vi "Main.vi"() -> ()   [LabVIEW 2019]
panel:
  out "Main Tabs":T1(tab)
  in  "START GAME":bool
  in  "EXPERT SELECT":bool
  in  "HARD SELECT":bool
  in  "MEDIUM SELECT":bool
  in  "EASY SELECT":bool
  in  "EASY CODE":T2
  in  "SUBMIT EASY CODE":bool
  in  "MEDIUM CODE":T3
  in  "SUBMIT MEDIUM CODE":bool
  in  "HARD CODE":T3
  in  "SUBMIT HARD CODE":bool
  in  "EXPERT CODE":cluster{"A":u8, "B":u8, "C":u8, "D":u8}
  in  "SUBMIT EXPERT CODE":bool
  # "You have 5 minutes to solve a puzzle and escape.\nSelect your difficulty below:"
  # "Using the items on the table to your left\nfind and enter the code below"
  # "Solve the puzzle on the table to your right\nto find the code to escape"
  # "Interpret my speech with the key from the walls to open the codex.\nThen go to the table behind you to enter my song below"
  # "Use the panels around the room to tell me\nwhat number each letter represents"
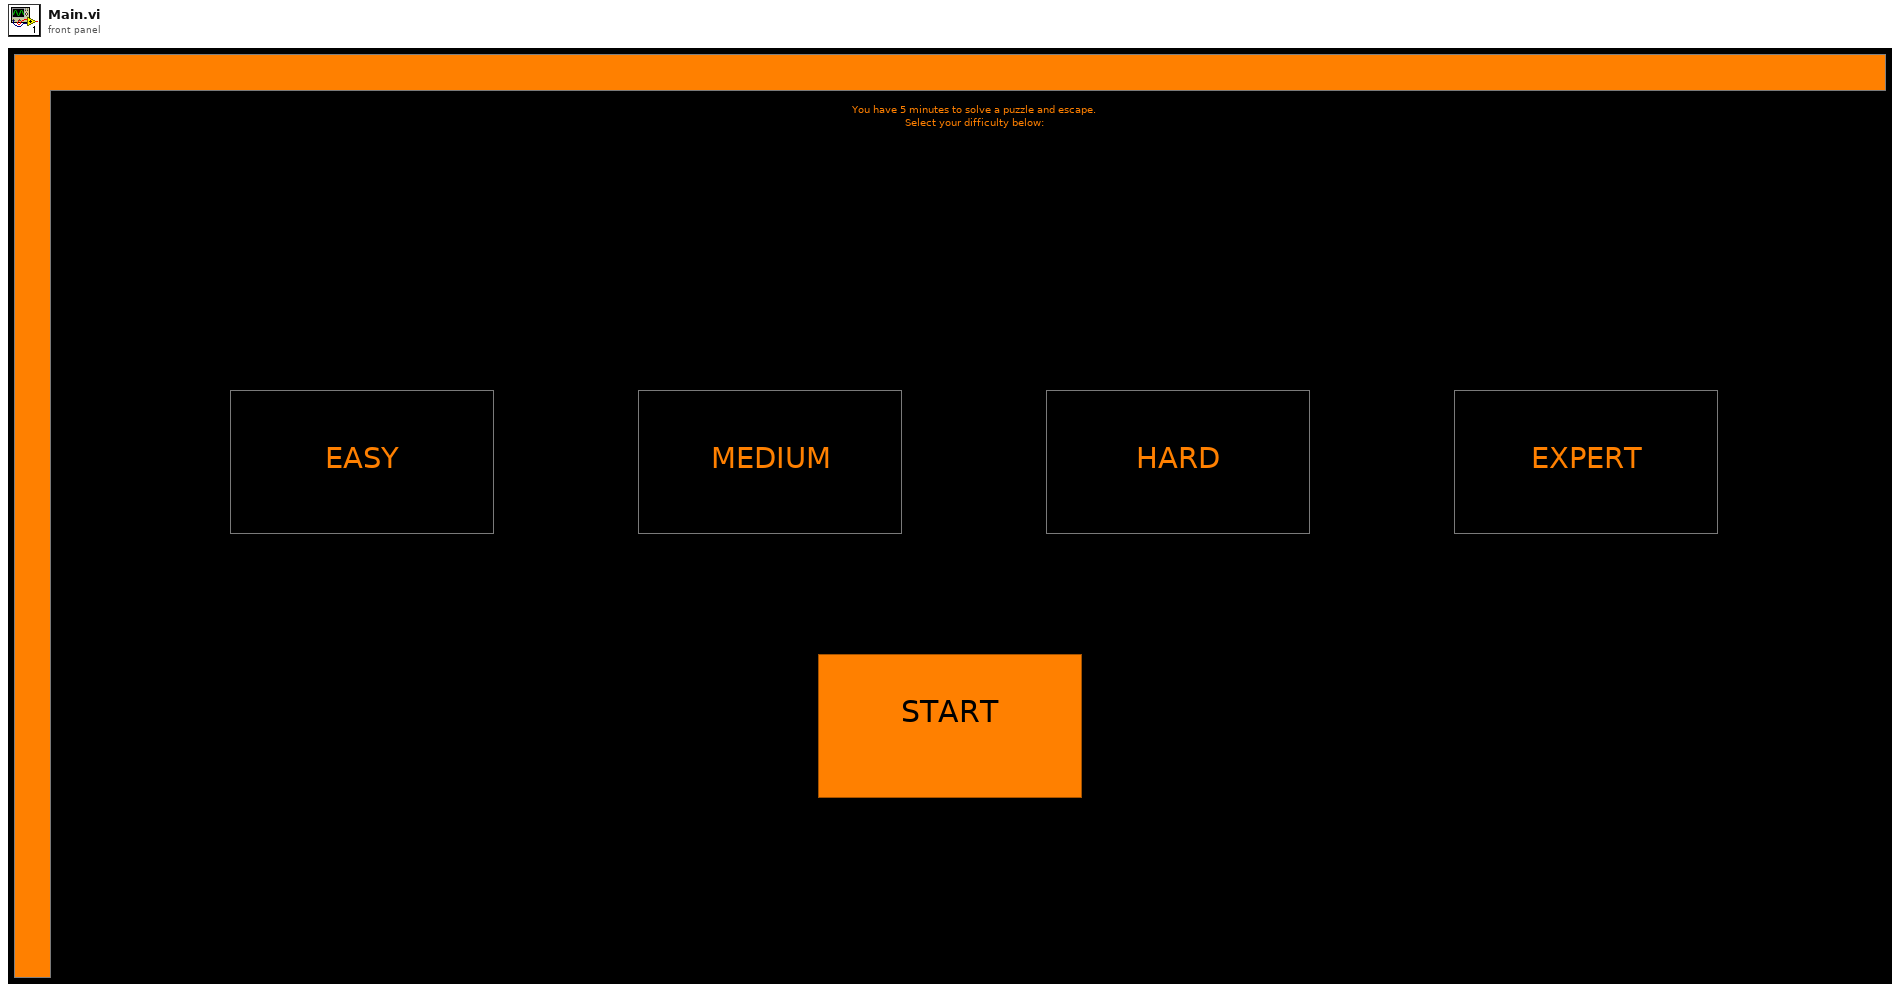
[diagram p1: front panel]
types:
  T1 = enum32{"START", "EASY", "MEDIUM", "HARD", "EXPERT", "END"}
  T2 = cluster{"CRANK":u8, "UV":u8, "MAZE":u8, "SCALE":u8}
  T3 = cluster{"DIGIT 1":u8, "DIGIT 2":u8, "DIGIT 3":u8, "DIGIT 4":u8}
  T4 = enum16{"INIT", "WAIT TO START", "GAME", "RESET", "END"}
  T5 = cluster{"CRANK":bool, "UV":bool, "MAZE":bool, "SCALE":bool}
  T6 = cluster{"DIGIT 1":bool, "DIGIT 2":bool, "DIGIT 3":bool, "DIGIT 4":bool}
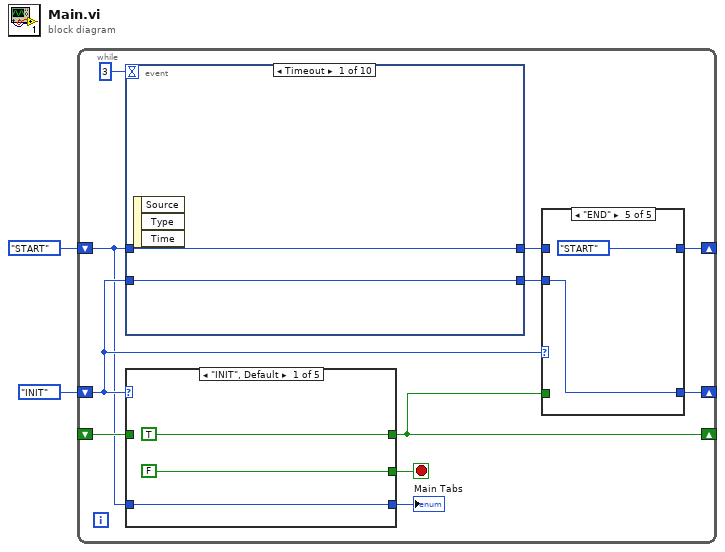
[diagram p0: block diagram]
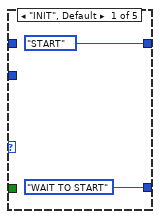
[diagram p2: hidden frame]
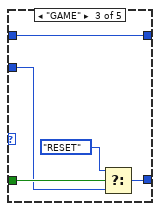
[diagram p4: hidden frame]
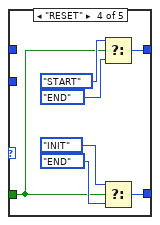
[diagram p5: hidden frame]
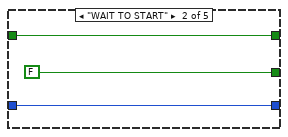
[diagram p6: hidden frame]
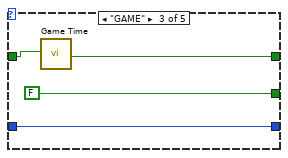
[diagram p7: hidden frame]
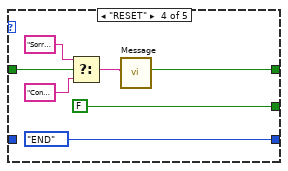
[diagram p8: hidden frame]
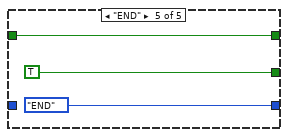
[diagram p9: hidden frame]
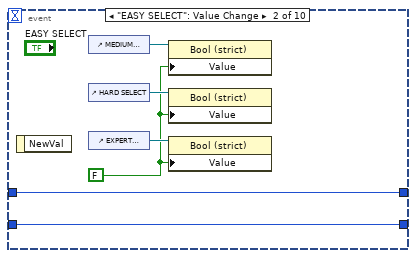
[diagram p10: hidden frame]
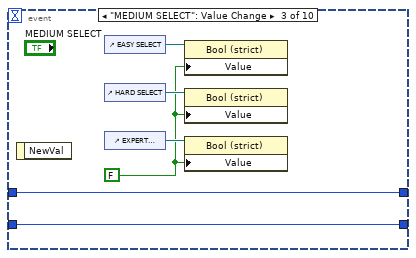
[diagram p11: hidden frame]
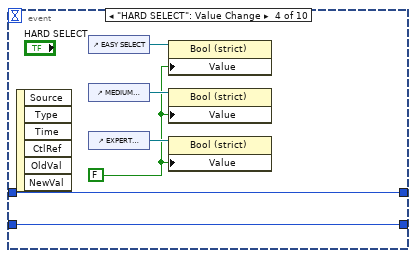
[diagram p12: hidden frame]
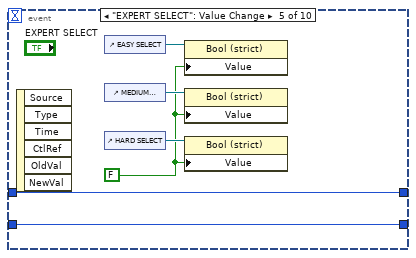
[diagram p13: hidden frame]
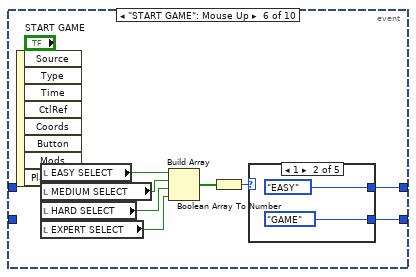
[diagram p14: hidden frame]
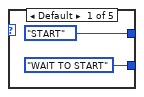
[diagram p15: hidden frame]
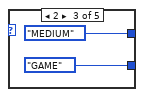
[diagram p16: hidden frame]
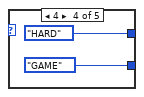
[diagram p17: hidden frame]
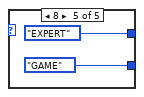
[diagram p18: hidden frame]
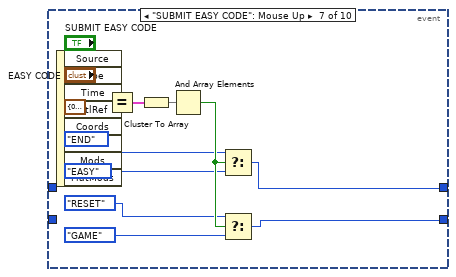
[diagram p19: hidden frame]
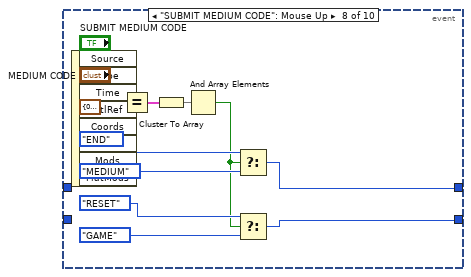
[diagram p20: hidden frame]
diagram:
  n1 = while {
    shift-right: [w3] -> _
    shift-left: T1."START" ("Main Tabs") -> [w6]
    shift-right: [w10] -> _
    shift-left: T4."INIT" -> [w12]
    shift-right: [w9] -> _
    shift-left: _ -> [w8]
    stop <- w5 stop-if-true
    n2 = event shown="[0] Timeout" {
      selector: _ -> [_ _ _ _ _ _ _ _ _ _]
      dyn-events: _ -> [_ _ _ _ _ _ _ _ _ _]
      timeout: 3 -> [_ _ _ _ _ _ _ _ _ _]
      tunnel: [w53 w55 w61 w67 w74 w79 w100 w108 w119 w130] -> w4
      tunnel: w6 -> [w53 w55 w61 w67 w74 _ _ _ _ _]
      tunnel: w12 -> [w52 w54 w60 w66 w73 _ _ _ _ _]
      tunnel: [w52 w54 w60 w66 w73 w78 w96 w107 w118 w129] -> w11
      event Timeout {
        n3 = event-data() -> ()  [unwired: 1 in, 3 out]
      }
      event "EASY SELECT": Value Change {
        w56 = FALSE ("Value")
        n4 = event-data() -> ()  [unwired: 1 in, 1 out]
        n5 = control-ref of="MEDIUM SELECT"() -> (w59:refnum<vi>)
        n6 = control-ref of="HARD SELECT"() -> (w58:refnum<vi>)
        n7 = control-ref of="EXPERT SELECT"() -> (w57:refnum<vi>)
        n8 = property class="Bool (strict)"(reference=w59, "Value"=w56) -> ()  [unwired: 1 in, 2 out]
        n9 = property class="Bool (strict)"(reference=w58, "Value"=w56) -> ()  [unwired: 1 in, 2 out]
        n10 = property class="Bool (strict)"(reference=w57, "Value"=w56) -> ()  [unwired: 1 in, 2 out]
      }
      event "MEDIUM SELECT": Value Change {
        w62 = FALSE ("Value")
        n11 = event-data() -> ()  [unwired: 1 in, 1 out]
        n12 = control-ref of="EASY SELECT"() -> (w65:refnum<vi>)
        n13 = control-ref of="HARD SELECT"() -> (w64:refnum<vi>)
        n14 = control-ref of="EXPERT SELECT"() -> (w63:refnum<vi>)
        n15 = property class="Bool (strict)"(reference=w65, "Value"=w62) -> ()  [unwired: 1 in, 2 out]
        n16 = property class="Bool (strict)"(reference=w64, "Value"=w62) -> ()  [unwired: 1 in, 2 out]
        n17 = property class="Bool (strict)"(reference=w63, "Value"=w62) -> ()  [unwired: 1 in, 2 out]
      }
      event "HARD SELECT": Value Change {
        w68 = FALSE ("Value")
        n18 = event-data() -> ()  [unwired: 1 in, 6 out]
        n19 = control-ref of="EASY SELECT"() -> (w71:refnum<vi>)
        n20 = control-ref of="MEDIUM SELECT"() -> (w70:refnum<vi>)
        n21 = control-ref of="EXPERT SELECT"() -> (w69:refnum<vi>)
        n22 = property class="Bool (strict)"(reference=w71, "Value"=w68) -> ()  [unwired: 1 in, 2 out]
        n23 = property class="Bool (strict)"(reference=w70, "Value"=w68) -> ()  [unwired: 1 in, 2 out]
        n24 = property class="Bool (strict)"(reference=w69, "Value"=w68) -> ()  [unwired: 1 in, 2 out]
      }
      event "EXPERT SELECT": Value Change {
        w72 = FALSE ("Value")
        n25 = event-data() -> ()  [unwired: 1 in, 6 out]
        n26 = control-ref of="EASY SELECT"() -> (w77:refnum<vi>)
        n27 = control-ref of="MEDIUM SELECT"() -> (w76:refnum<vi>)
        n28 = control-ref of="HARD SELECT"() -> (w75:refnum<vi>)
        n29 = property class="Bool (strict)"(reference=w77, "Value"=w72) -> ()  [unwired: 1 in, 2 out]
        n30 = property class="Bool (strict)"(reference=w76, "Value"=w72) -> ()  [unwired: 1 in, 2 out]
        n31 = property class="Bool (strict)"(reference=w75, "Value"=w72) -> ()  [unwired: 1 in, 2 out]
      }
      event "START GAME": Mouse Up {
        n32 = event-data() -> ()  [unwired: 1 in, 8 out]
        n33 = local read "EASY SELECT"() -> (w85:bool)
        n34 = local read "MEDIUM SELECT"() -> (w82:bool)
        n35 = local read "HARD SELECT"() -> (w84:bool)
        n36 = local read "EXPERT SELECT"() -> (w83:bool)
        n37 = Build Array(w85, w82, w84, w83) -> (w81:bool[])
        n38 = Boolean Array To Number(Boolean array=w81) -> (number=w80:u32)
        n39 = case shown="1" w80 {
          tunnel: [T1."START" ("Main Tabs") T1."EASY" ("Main Tabs") T1."MEDIUM" ("Main Tabs") T1."HARD" ("Main Tabs") T1."EXPERT" ("Main Tabs")] -> w79
          tunnel: [T4."WAIT TO START" T4."GAME" T4."GAME" T4."GAME" T4."GAME"] -> w78
          frame Default {
          }
          frame 1 {
          }
          frame 2 {
          }
          frame 4 {
          }
          frame 8 {
          }
        }
      }
      event "SUBMIT EASY CODE": Mouse Up {
        n40 = event-data() -> ()  [unwired: 1 in, 8 out]
        n41 = Equal?(x="EASY CODE", y=T2 {"CRANK"=0, "UV"=0, "MAZE"=0, "SCALE"=0}) -> (x = y?=w104:T5)
        n42 = Cluster To Array(cluster=w104) -> (array=w103:bool[])
        n43 = And Array Elements(Boolean array=w103) -> (logical AND=w102:bool)
        n44 = Select(t=T1."END" ("Main Tabs"), s=w102, f=T1."EASY" ("Main Tabs")) -> (s? t:f=w100:T1)
        n45 = Select(t=T4."RESET", s=w102, f=T4."GAME") -> (s? t:f=w96:T4)
      }
      event "SUBMIT MEDIUM CODE": Mouse Up {
        n46 = event-data() -> ()  [unwired: 1 in, 8 out]
        n47 = Equal?(x="MEDIUM CODE", y=T3 {"DIGIT 1"=0, "DIGIT 2"=0, "DIGIT 3"=0, "DIGIT 4"=0}) -> (x = y?=w117:T6)
        n48 = Cluster To Array(cluster=w117) -> (array=w116:bool[])
        n49 = And Array Elements(Boolean array=w116) -> (logical AND=w109:bool)
        n50 = Select(t=T1."END" ("Main Tabs"), s=w109, f=T1."MEDIUM" ("Main Tabs")) -> (s? t:f=w108:T1)
        n51 = Select(t=T4."RESET", s=w109, f=T4."GAME") -> (s? t:f=w107:T4)
      }
      event "SUBMIT HARD CODE": Mouse Up {
        n52 = event-data() -> ()  [unwired: 1 in, 8 out]
        n53 = Equal?(x="HARD CODE", y=T3 {"DIGIT 1"=0, "DIGIT 2"=0, "DIGIT 3"=0, "DIGIT 4"=0}) -> (x = y?=w128:T6)
        n54 = Cluster To Array(cluster=w128) -> (array=w127:bool[])
        n55 = And Array Elements(Boolean array=w127) -> (logical AND=w122:bool)
        n56 = Select(t=T1."END" ("Main Tabs"), s=w122, f=T1."MEDIUM" ("Main Tabs")) -> (s? t:f=w119:T1)
        n57 = Select(t=T4."RESET", s=w122, f=T4."GAME") -> (s? t:f=w118:T4)
      }
      event "SUBMIT EXPERT CODE": Mouse Up {
        n58 = event-data() -> ()  [unwired: 1 in, 8 out]
        n59 = Equal?(x="EXPERT CODE", y=cluster{"A":u8, "B":u8, "C":u8, "D":u8} {"A"=0, "B"=0, "C"=0, "D"=0}) -> (x = y?=w139:cluster{"A":bool, "B":bool, "C":bool, "D":bool})
        n60 = Cluster To Array(cluster=w139) -> (array=w138:bool[])
        n61 = And Array Elements(Boolean array=w138) -> (logical AND=w133:bool)
        n62 = Select(t=T1."END" ("Main Tabs"), s=w133, f=T1."MEDIUM" ("Main Tabs")) -> (s? t:f=w130:T1)
        n63 = Select(t=T4."RESET", s=w133, f=T4."GAME") -> (s? t:f=w129:T4)
      }
    }
    n64 = case shown="\"INIT\", Default" w12 {
      tunnel: [TRUE ("Time has Elapsed") w36 w41 w46 w49] -> w9
      tunnel: w8 -> [_ w36 w39 w45 w49]
      tunnel: [w33 w37 w40 T1."END" ("Main Tabs") T1."END" ("Main Tabs")] -> w7
      tunnel: w6 -> [w33 w37 w40 _ _]
      tunnel: [FALSE FALSE FALSE FALSE TRUE] -> w5
      frame "INIT", Default {
      }
      frame "WAIT TO START" {
      }
      frame "GAME" {
        n65 = call "Game Time"("Reset"=w39) -> ("Time has Elapsed"=w41:bool)  [unwired: 11 in, 7 out]
      }
      frame "RESET" {
        n66 = Select(t="Sorry you ran out of time. \nReset the room for another group?", s=w45, f="Congrats on escaping! \nReset the room for another group?") -> (s? t:f=w42:string)
        n67 = call "Message"("Message"=w42) -> ("Yes"=w46:bool)  [unwired: 9 in, 1 out]
      }
      frame "END" {
      }
    }
    "Main Tabs" <- w7
    n68 = case shown="\"END\"" w12 {
      tunnel: w11 -> [_ w17 w19 _ w31]
      tunnel: [T4."WAIT TO START" w17 w20 w27 w31] -> w10
      tunnel: w9 -> [_ _ w22 w23 _]
      tunnel: w4 -> [_ w16 w18 _ _]
      tunnel: [T1."START" ("Main Tabs") w16 w18 w26 T1."START" ("Main Tabs")] -> w3
      frame "INIT", Default {
      }
      frame "WAIT TO START" {
      }
      frame "GAME" {
        n69 = Select(t=T4."RESET", s=w22, f=w19) -> (s? t:f=w20:T4)
      }
      frame "RESET" {
        n70 = Select(t=T1."START" ("Main Tabs"), s=w23, f=T1."END" ("Main Tabs")) -> (s? t:f=w26:T1)
        n71 = Select(t=T4."INIT", s=w23, f=T4."END") -> (s? t:f=w27:T4)
      }
      frame "END" {
      }
    }
  }
